vi "CTRE_Phoenix_CANcoder_SetPositionToAbsolute.vi"(6 "timeoutMs":u32, 8 "error in (no error)":errorcluster, 11 "CTRE_CANcoder_DeviceRef":T1) -> (0 "error out":errorcluster, 3 "CTRE_CANcoder_DeviceRef":T1)   [LabVIEW 2020]
doc: "Sets the position of the sensor to match the magnet's \"Absolute Sensor\".\nThe units are determined by the coefficient and unit-string configuration params, default is degrees."
uses:
  <vilib>/Rock Robotics/WPI/ThirdParty/Phoenix-LabVIEW/CANCoder/Controls/CTRE_Phoenix_CANcoder_DeviceRef.ctl
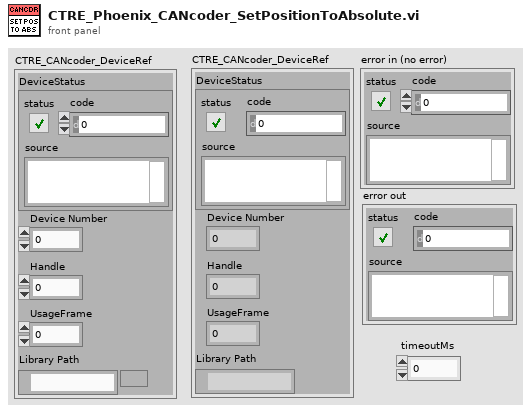
[diagram p1: front panel]
types:
  T1 = typedef "CTRE_Phoenix_CANcoder_DeviceRef.ctl" = cluster{"DeviceStatus":errorcluster, "Device Number":u8, "Handle":u64, "UsageFrame":u32, "Library Path":path}
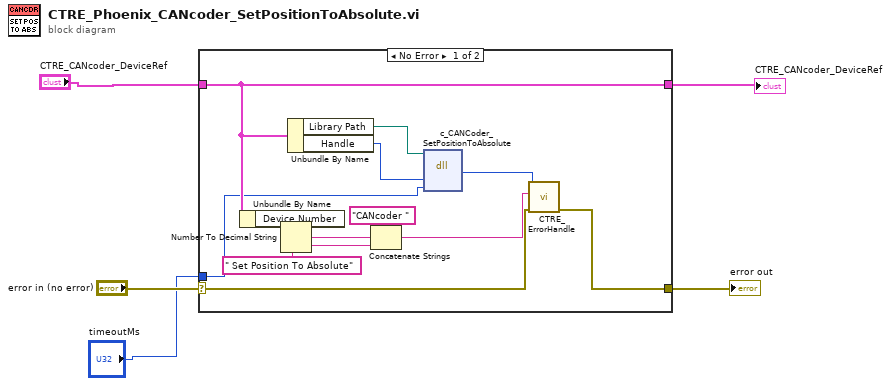
[diagram p0: block diagram]
diagram:
  n1 = case shown="No Error" "error in (no error)" {
    selector: "error in (no error)" -> [w8 w18]
    tunnel: [w7 w18] -> w4
    tunnel: [w10 w19] -> w1
    tunnel: "CTRE_CANcoder_DeviceRef" -> [w10 w19]
    tunnel: "timeoutMs" -> [w6 _]
    frame No Error {
      n2 = Unbundle By Name(w10) -> ("Device Number"=w14:u8)
      n3 = Number To Decimal String(number=w14) -> (decimal integer string=w13:string)  [unwired: 1 in]
      n4 = Unbundle By Name(w10) -> ("Library Path"=w17:path, "Handle"=w16:u64)
      n5 = Concatenate Strings("CANcoder " ("string"), w13, " Set Position To Absolute" ("string")) -> (w9:string)
      n6 = dll-call lib="?" fn="c_CANCoder_SetPositionToAbsolute"(path in=w17, "handle"=w16, "timeoutms"=w6) -> ("return type"=w15:i32)  [unwired: 4 in, 2 out]
      n7 = call <vilib>:"CTRE_ErrorHandle.vi"("error in"=w8, "origin"=w9, "code"=w15) -> ("error out"=w7:errorcluster)  [unwired: 8 in]
    }
    frame Error {
    }
  }
  "error out" <- w4
  "CTRE_CANcoder_DeviceRef" <- w1
